vi "P612CW.vi"(4 "Special Function In":string, 6 "Velocity":dbl, 7 "Abort":bool, 8 "Axis":bool[](array[boolean]), 9 "Positions":dbl[](array[numeric]), 10 "Action":T1=enum."MVR", 11 "VISA In":refnum<visa-resource-name>) -> (0 "Special Function":string, 1 "Status":bool, 2 "Position Out":dbl[](array[numeric]), 3 "VISA Out":refnum<visa-resource-name>)   [LabVIEW 2014]
uses:
  Controls/StageStates.ctl
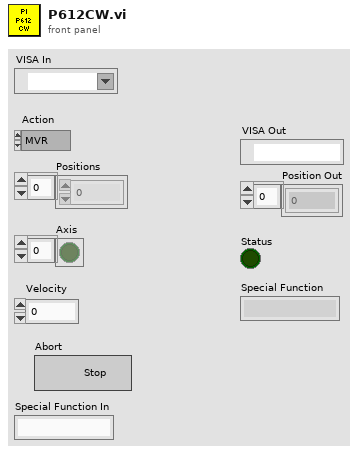
[diagram p1: front panel]
types:
  T1 = typedef "StageStates.ctl" = enum16{"POSITION", "MVR", "MOVE", "HALT", "ONTARGET", "ERROR", "EXIT", "HOME", "ZEROPOS", "NANOPOS", "QUIT", "ANALOG"}
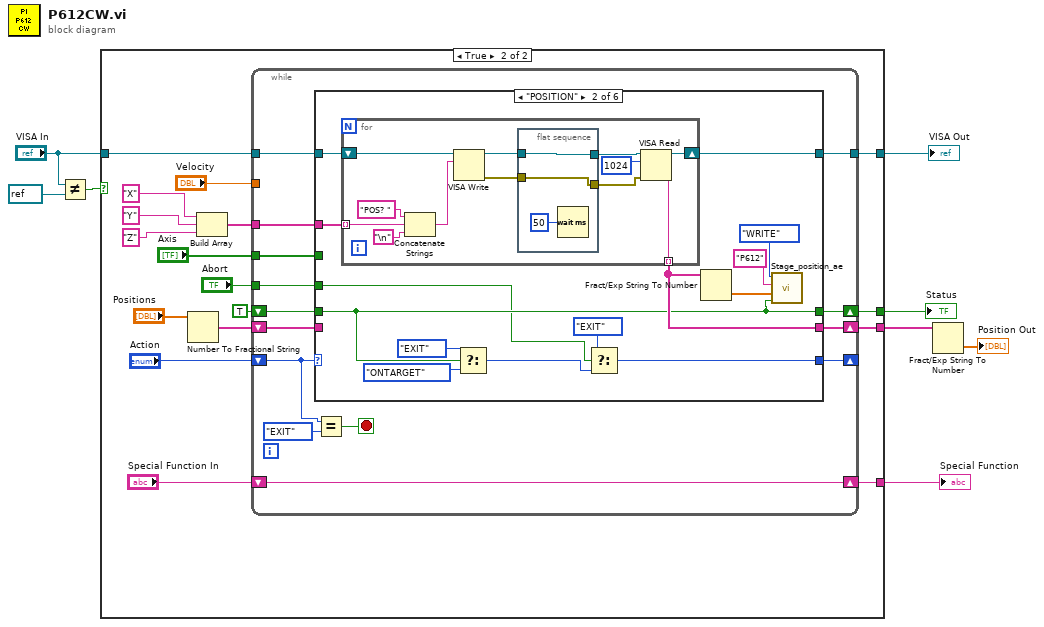
[diagram p0: block diagram]
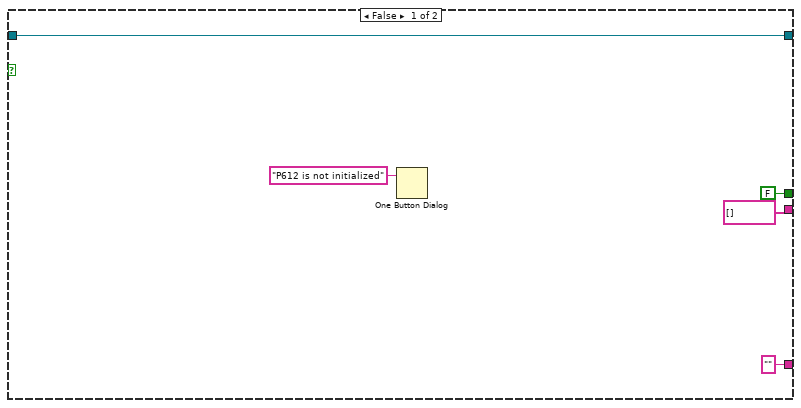
[diagram p2: hidden frame]
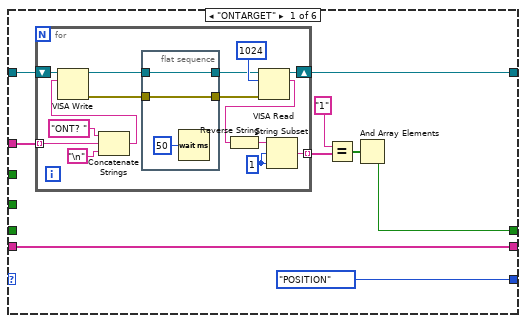
[diagram p3: hidden frame]
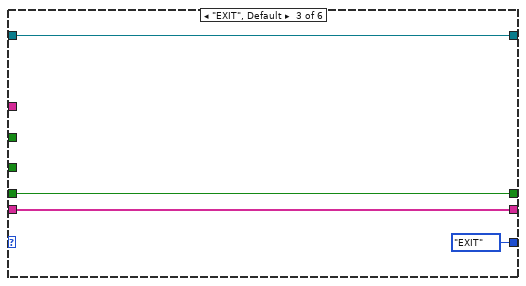
[diagram p4: hidden frame]
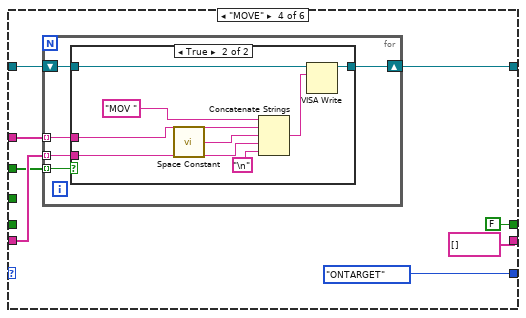
[diagram p5: hidden frame]
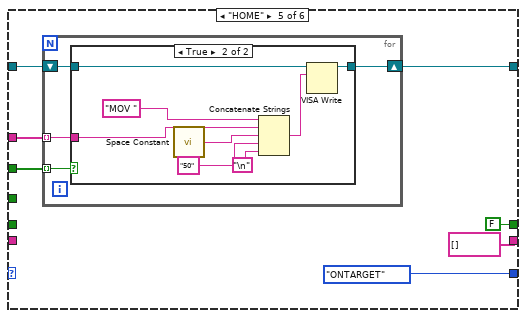
[diagram p7: hidden frame]
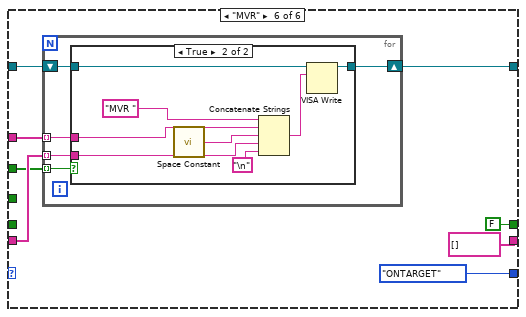
[diagram p9: hidden frame]
diagram:
  n1 = Not Equal?(x="VISA In", y=refnum<visa-resource-name> refnum ("VISA In")) -> (x != y?=w8:bool)
  n2 = case shown="True" w8 {
    tunnel: "VISA In" -> [w12 w30]
    tunnel: [w12 w19] -> w5
    tunnel: [FALSE w18] -> w3
    tunnel: [string[] [] w17] -> w2
    tunnel: ["" ("Special Function In") w16] -> w1
    frame False {
      n3 = One Button Dialog(message="P612 is not initialized") -> ()  [unwired: 1 in, 1 out]
    }
    frame True {
      n4 = Number To Fractional String(number="Positions") -> (F-format string=w23:string[])  [unwired: 3 in]
      n5 = Build Array("X", "Y", "Z") -> (w26:string[])
      n6 = while {
        tunnel: w26 -> [w44]
        tunnel: w30 -> [w43]
        shift-right: [w35] -> _
        shift-left: "Action" -> [w38]
        shift-right: [w41] -> w17
        shift-left: w23 -> [w42]
        shift-right: [w39] -> w18
        shift-left: TRUE -> [w40]
        tunnel: "Axis" -> [w37]
        shift-right: [w34] -> w16
        shift-left: "Special Function In" -> [w34]
        tunnel: "Velocity" -> [_]
        tunnel: [w33] -> w19
        tunnel: "Abort" -> [w31]
        stop <- w32 stop-if-true
        n7 = case shown="\"POSITION\"" w38 {
          tunnel: w44 -> [w53 w85 _ w112 w133 w154]
          tunnel: w43 -> [w47 w84 w104 w111 w132 w153]
          tunnel: w42 -> [w49 _ w102 w110 _ w152]
          tunnel: [w49 w74 w102 string[] [] string[] [] string[] []] -> w41
          tunnel: w40 -> [_ w73 w103 _ _ _]
          tunnel: [w48 w73 w103 FALSE FALSE FALSE] -> w39
          tunnel: w37 -> [_ _ _ w109 w131 w151]
          tunnel: [StageStates."POSITION" ("Action") w79 StageStates."EXIT" ("Action") StageStates."ONTARGET" ("Action") StageStates."ONTARGET" ("Action") StageStates."ONTARGET" ("Action")] -> w35
          tunnel: [w46 w78 w104 w107 w129 w149] -> w33
          tunnel: w31 -> [_ w72 _ _ _ _]
          frame "ONTARGET" {
            n8 = for {
              tunnel: w53 -> [w68] mode=indexing
              tunnel: [w67] -> w52 mode=indexing
              shift-right: [w58] -> w46
              shift-left: w47 -> [w59]
              w62 = 1 ("length (rest)")
              n9 = Concatenate Strings("ONT? " ("string"), w68, "\n") -> (w61:string)
              n10 = VISA Write(VISA resource name=w59, write buffer=w61) -> (VISA resource name out=w57:refnum<visa-resource-name>, error out=w54:errorcluster)  [unwired: 1 in, 1 out]
              n11 = flat-sequence {
                tunnel: w57 -> [w70]
                tunnel: [w70] -> w56
                tunnel: [w69] -> w55
                tunnel: w54 -> [w69]
                frame #0 {
                  n12 = Wait (ms)(milliseconds to wait=u32 50) -> ()  [unwired: 1 out]
                }
              }
              n13 = VISA Read(VISA resource name=w56, byte count=u32 1024, error in (no error)=w55) -> (VISA resource name out=w58:refnum<visa-resource-name>, read buffer=w60:string)  [unwired: 2 out]
              n14 = Reverse String(1:w60) -> (0:w63:string)
              n15 = String Subset(string=w63, offset (0)=w62, length (rest)=w62) -> (substring=w67:string)
            }
            n16 = Equal?(x="1", y=w52) -> (x = y?=w50:bool[])
            n17 = And Array Elements(Boolean array=w50) -> (logical AND=w48:bool)
          }
          frame "POSITION" {
            n18 = for {
              tunnel: w85 -> [w97] mode=indexing
              tunnel: [w91] -> w74 mode=indexing
              shift-right: [w86] -> w78
              shift-left: w84 -> [w92]
              n19 = Concatenate Strings("POS? " ("string"), w97, "\n") -> (w93:string)
              n20 = VISA Write(VISA resource name=w92, write buffer=w93) -> (VISA resource name out=w89:refnum<visa-resource-name>, error out=w87:errorcluster)  [unwired: 1 in, 1 out]
              n21 = flat-sequence {
                tunnel: [w100] -> w90
                tunnel: w89 -> [w100]
                tunnel: [w99] -> w88
                tunnel: w87 -> [w99]
                frame #0 {
                  n22 = Wait (ms)(milliseconds to wait=u32 50) -> ()  [unwired: 1 out]
                }
              }
              n23 = VISA Read(VISA resource name=w90, byte count=u32 1024, error in (no error)=w88) -> (VISA resource name out=w86:refnum<visa-resource-name>, read buffer=w91:string)  [unwired: 2 out]
            }
            n24 = Select(t=StageStates."EXIT" ("Action"), s=w73, f=StageStates."ONTARGET" ("Action")) -> (s? t:f=w82:T1)
            n25 = Select(t=StageStates."EXIT", s=w72, f=w82) -> (s? t:f=w79:T1)
            n26 = Fract/Exp String To Number(string=w74) -> (number=w77:dbl[])  [unwired: 3 in, 1 out]
            n27 = call "Stage_position_ae.vi"("Status In"=w73, "Position In"=w77, "StageID"="P612", "Enum"=enum16{"WRITE", "READ"}."WRITE") -> ()  [unwired: 6 in, 2 out]
          }
          frame "EXIT", Default {
          }
          frame "MOVE" {
            n28 = for {
              tunnel: w112 -> [w117] mode=indexing
              tunnel: w110 -> [w116] mode=indexing
              shift-right: [w114] -> w107
              shift-left: w111 -> [w115]
              tunnel: w109 -> [w113] mode=indexing
              n29 = case shown="True" w113 {
                tunnel: w117 -> [_ w124]
                tunnel: w116 -> [_ w121]
                tunnel: w115 -> [w118 w120]
                tunnel: [w118 w119] -> w114
                frame False {
                }
                frame True {
                  n30 = call <vilib>:"Space Constant.vi"() -> ("String"=w122:string)
                  n31 = Concatenate Strings("MOV ", w124, w122, w121, "\n") -> (w126:string)
                  n32 = VISA Write(VISA resource name=w120, write buffer=w126) -> (VISA resource name out=w119:refnum<visa-resource-name>)  [unwired: 1 in, 2 out]
                }
              }
            }
          }
          frame "HOME" {
            n33 = for {
              tunnel: w133 -> [w137] mode=indexing
              shift-right: [w135] -> w129
              shift-left: w132 -> [w136]
              tunnel: w131 -> [w134] mode=indexing
              n34 = case shown="True" w134 {
                tunnel: w137 -> [_ w144]
                tunnel: w136 -> [w138 w141]
                tunnel: [w138 w140] -> w135
                frame False {
                }
                frame True {
                  n35 = call <vilib>:"Space Constant.vi"() -> ("String"=w142:string)
                  n36 = Concatenate Strings("MOV ", w144, w142, "50" ("string"), "\n") -> (w146:string)
                  n37 = VISA Write(VISA resource name=w141, write buffer=w146) -> (VISA resource name out=w140:refnum<visa-resource-name>)  [unwired: 1 in, 2 out]
                }
              }
            }
          }
          frame "MVR" {
            n38 = for {
              tunnel: w154 -> [w159] mode=indexing
              tunnel: w152 -> [w158] mode=indexing
              shift-right: [w156] -> w149
              shift-left: w153 -> [w157]
              tunnel: w151 -> [w155] mode=indexing
              n39 = case shown="True" w155 {
                tunnel: w159 -> [_ w166]
                tunnel: w158 -> [_ w163]
                tunnel: w157 -> [w160 w162]
                tunnel: [w160 w161] -> w156
                frame False {
                }
                frame True {
                  n40 = call <vilib>:"Space Constant.vi"() -> ("String"=w164:string)
                  n41 = Concatenate Strings("MVR ", w166, w164, w163, "\n") -> (w168:string)
                  n42 = VISA Write(VISA resource name=w162, write buffer=w168) -> (VISA resource name out=w161:refnum<visa-resource-name>)  [unwired: 1 in, 2 out]
                }
              }
            }
          }
        }
        n43 = Equal?(x=w38, y=StageStates."EXIT") -> (x = y?=w32:bool)
      }
    }
  }
  "VISA Out" <- w5
  "Status" <- w3
  "Special Function" <- w1
  n44 = Fract/Exp String To Number(string=w2) -> (number=→"Position Out":dbl[])  [unwired: 3 in, 1 out]
